vi "CVT Double IndexRead.vi"(3 "error in (no error)":errorcluster, 5 "Tag Index":i32) -> (0 "error out":errorcluster, 1 "Value":dbl)   [LabVIEW 2016]
uses:
  <vilib>/NI/Current Value Table/DataTypes/Double_Read Index.vi
  <vilib>/NI/Current Value Table/Memory Block.vi
  <vilib>/NI/Current Value Table/DataTypes/Double_Memory Block.vi
  <vilib>/NI/Current Value Table/Current Value Table.lvlib
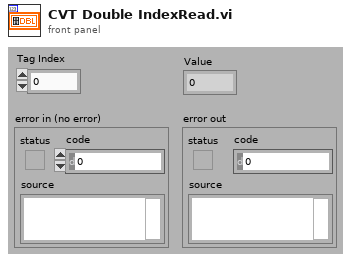
[diagram p1: front panel]
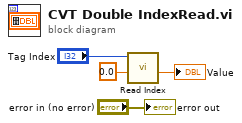
[diagram p0: block diagram]
diagram:
  n1 = call-poly <vilib>:"Read Index.vi"("Default"=0.0, "Index"="Tag Index") -> ("Value"=→"Value":dbl)  [unwired: 9 in]
  "error out" <- "error in (no error)"
